vi "Search Label Array for Index of Label.vi"(6 "Label Map":i32[](array[numeric]), 8 "error in (no error)":errorcluster, 9 "sdi":u32, 10 "label":u32) -> (0 "error out":errorcluster, 1 "Label Found?":bool, 3 "Index":i32)   [LabVIEW 2011, in "AIT 1553 Custom Device.lvlib"]
uses:
  AIT 1553 Custom Device.lvlib
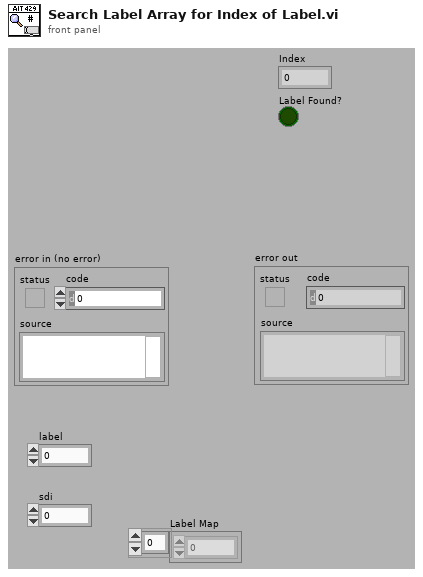
[diagram p1: front panel]
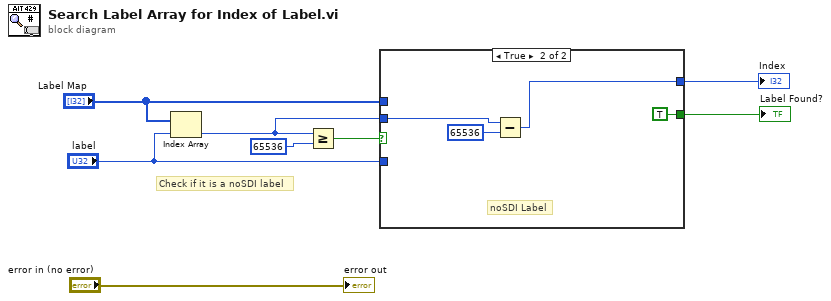
[diagram p0: block diagram]
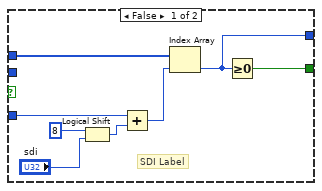
[diagram p2: hidden frame]
diagram:
  # "Check if it is a noSDI label"
  n1 = Index Array(array="Label Map", index="label") -> (element=w1:i32)
  n2 = Greater Or Equal?(x=w1, y=65536) -> (x >= y?=w2:bool)
  n3 = case shown="True" w2 {
    tunnel: "Label Map" -> [w16 _]
    tunnel: [w15 w17] -> w7
    tunnel: [w14 TRUE] -> w6
    tunnel: "label" -> [w10 _]
    tunnel: w1 -> [_ w19]
    frame False {
      # "SDI Label"
      n4 = Logical Shift(y=i8 8, x="sdi") -> (x << y=w11:u32)
      n5 = Add(x=w10, y=w11) -> (x+y=w9:u32)
      n6 = Index Array(array=w16, index=w9) -> (element=w15:i32)
      n7 = Greater Or Equal To 0?(x=w15) -> (x >= 0?=w14:bool)
    }
    frame True {
      # "noSDI Label"
      n8 = Subtract(x=w19, y=65536) -> (x-y=w17:i32)
    }
  }
  "Index" <- w7
  "Label Found?" <- w6
  "error out" <- "error in (no error)"
